vi "Handle Error.vi"(8 "error in (no error)":errorcluster, 11 "CS++DeviceActor in":refnum<class "CS++DeviceActor.lvclass">) -> (0 "error out":errorcluster, 2 "stop actor?":bool=TRUE, 3 "CS++DeviceActor out":refnum<class "CS++DeviceActor.lvclass">)   [LabVIEW 2016, in "CS++DeviceActor.lvlib" / "CS++DeviceActor.lvclass"]
doc: "(<B>Filename</B>: Actor Framework.lvlib:Actor.lvclass:Handle Error.vi)\n\nDefines how the actor handles an error that occurred while processing a message.\n\nBy default, this method does nothing except stop the actor. This method also treats error code 43 (coming from <B>error in</B>) as a sign that the actor shut down normally. In this situation, the Handle Error method does not return the error on <B>error out</B>, meaning the actor's caller will not receive it. All other error codes will be returned on <B>error out</B>.\n\nA descendant class may override this method to change this behavior."
uses:
  CS++DeviceActor.lvclass
  CS++BaseActor/CS++BaseActor.lvclass
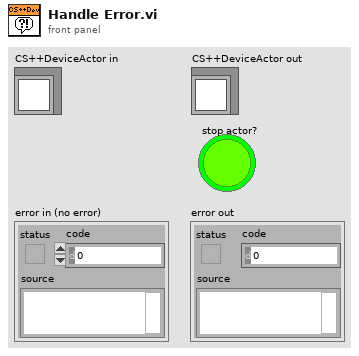
[diagram p1: front panel]
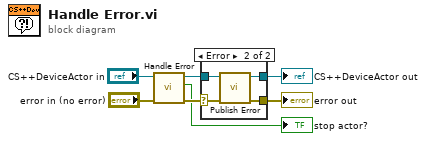
[diagram p0: block diagram]
diagram:
  n1 = call-parent "Handle Error.vi"("error in (no error)"="error in (no error)", "CS++BaseActor in"="CS++DeviceActor in") -> ("error out"=w5:errorcluster, "stop actor?"=→"stop actor?":bool, "CS++BaseActor out"=w4:refnum<class "CS++DeviceActor.lvclass">)  [unwired: 7 in]
  n2 = case shown="Error" w5 {
    selector: w5 -> [w8 w13]
    tunnel: w4 -> [w9 w12]
    tunnel: [w9 w11] -> w3
    tunnel: [w8 w10] -> w2
    frame No Error {
    }
    frame Error {
      n3 = call "Publish Error.vi"("error in (no error)"=w13, "CS++DeviceActor in"=w12) -> ("error out"=w10:errorcluster, "CS++DeviceActor out"=w11:refnum<class "CS++DeviceActor.lvclass">)  [unwired: 8 in]
    }
  }
  "CS++DeviceActor out" <- w3
  "error out" <- w2
